vi "Get Interrupt Status.vi"(7 "I2C Channel":u8, 8 "error in (no error)":errorcluster, 11 "LINX Resource In":T1) -> (0 "error out":errorcluster, 1 "Raw Data Ready":bool, 2 "PLL Ready":bool, 3 "LINX Resource Out":T1)   [LabVIEW 2014, in "LMH-LINX.lvlib" / "ITG3200.lvlib"]
uses:
  <vilib>/MakerHub/LINX/Public/Sensors/Gyroscopes/ITG3200/ITG3200.lvlib
  <vilib>/MakerHub/LINX/Private/Type Defs/LINX Ref.ctl
  <vilib>/MakerHub/LINX/Private/Type Defs/Platform.ctl
  <vilib>/MakerHub/LINX/Private/Type Defs/Interface.ctl
  <vilib>/MakerHub/LINX/Private/Device/Type Defs/LINX Device Config.ctl
  <vilib>/MakerHub/LINX/Private/Device/Type Defs/TCP Config.ctl
  <vilib>/MakerHub/LINX/Private/Device/Type Defs/Channels.ctl
  <vilib>/MakerHub/LINX/Private/Local IO/LinxI2cWrite.vi
  <vilib>/MakerHub/LINX/Public/Utilities/Check Channel.vi
  <vilib>/MakerHub/LINX/Private/Utilties/Generate Error.vi
  <vilib>/MakerHub/LINX/LMH-LINX.lvlib
  <vilib>/MakerHub/LINX/Private/Device/Device.lvlib
panel:
  # "INPUTS"
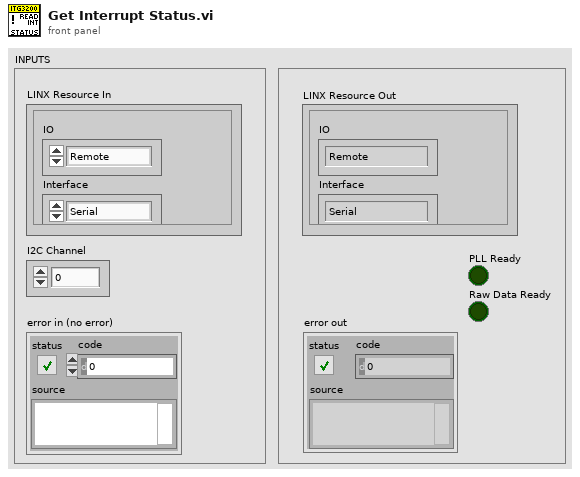
[diagram p1: front panel]
types:
  T1 = typedef "LMH-LINX.lvlib/LINX Ref.ctl" = cluster{"IO":T2, "Interface":T3, "LINX Device Config":T4}
  T2 = typedef "LMH-LINX.lvlib/Platform.ctl" = enum16{"Remote", "Local"}
  T3 = typedef "LMH-LINX.lvlib/Interface.ctl" = enum16{"Serial", "TCP"}
  T4 = typedef "LMH-LINX.lvlib/Device.lvlib/LINX Device Config.ctl" = cluster{"Interface":T3, "COM Port":refnum<visa-resource-name>, "TCP Configuration":T5, "Device Family":u8, "Device ID":u8, "Device Name":string, "TCP Ref":refnum<k5>, "Channels":T6}
  T5 = typedef "LMH-LINX.lvlib/Device.lvlib/TCP Config.ctl" = cluster{"IP Address":string, "Port":u16}
  T6 = typedef "LMH-LINX.lvlib/Channels.ctl" = cluster{"DI":u8[], "DO":u8[], "AI":u8[], "AO":u8[], "PWM":u8[], "QE":u8[], "UART":u8[], "I2C 2":u8[], "SPI":u8[], "CAN":u8[], "Servo":u8[], "AI Ref (V)":dbl, "AI Resolution (Bits)":u8, "AO Ref (V)":dbl, "AO Resolution (Bits)":u8}
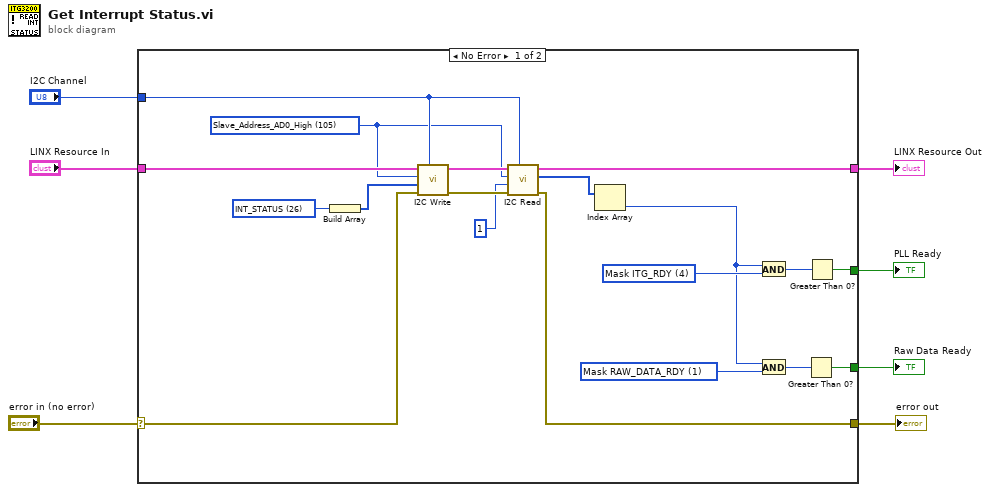
[diagram p0: block diagram]
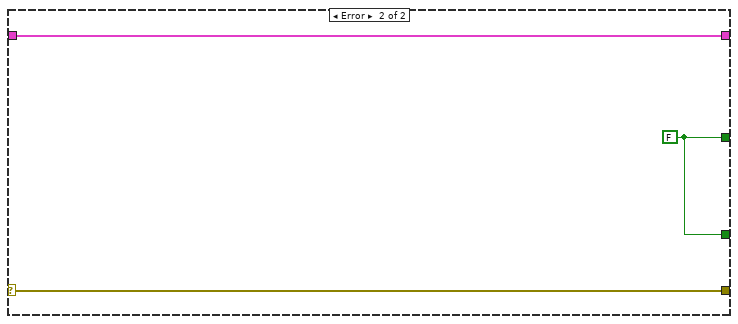
[diagram p2: hidden frame]
diagram:
  n1 = case shown="No Error" "error in (no error)" {
    selector: "error in (no error)" -> [w25 w29]
    tunnel: [w24 w29] -> w6
    tunnel: "LINX Resource In" -> [w26 w28]
    tunnel: "I2C Channel" -> [w22 _]
    tunnel: [w23 w28] -> w3
    tunnel: [w9 w27] -> w2
    tunnel: [w8 w27] -> w1
    frame No Error {
      w13 = u8 1 items=["Mask ITG_RDY"=4, "Mask RAW_DATA_RDY"=1] ("<INT STATUS> Register Masks")
      w14 = u8 4 items=["Mask ITG_RDY"=4, "Mask RAW_DATA_RDY"=1] ("<INT STATUS> Register Masks")
      w21 = u8 26 items=["WHO_AM_I"=0, "SMPLRT_DIV"=21, "DLPF_FS"=22, "INT_CFG"=23, "INT_STATUS"=26, "TEMP_OUT_H"=27, "TEMP_OUT_L"=28, "GYRO_XOUT_H"=29, "GYRO_XOUT_L"=30, "GYRO_YOUT_H"=31, "GYRO_YOUT_L"=32, "GYRO_ZOUT_H"=33, "GYRO_ZOUT_L"=34, "PWR_MGM"=62] ("Register Map")
      w17 = u8 105 items=["Slave_Address_AD0_Low"=104, "Slave_Address_AD0_High"=105] ("Slave Addresses")
      n2 = Build Array(w21) -> (w20:u8[])
      n3 = call <vilib>:"I2C Write.vi"("I2C Channel"=w22, "Error In"=w25, "Data"=w20, "I2C Slave Address (0)"=w17, "LINX Resource"=w26) -> ("Error Out"=w18:errorcluster, "LINX Resource"=w19:T1)  [unwired: 5 in]
      n4 = call <vilib>:"I2C Read.vi"("I2C Channel"=w22, "Error In"=w18, "Bytes To Read"=u8 1, "I2C Slave Address (0)"=w17, "LINX Resource"=w19) -> ("Error Out"=w24:errorcluster, "Data"=w15:u8[], "LINX Resource"=w23:T1)  [unwired: 4 in]
      n5 = Index Array(array=w15) -> (element=w12:u8)  [unwired: 1 in]
      n6 = And(x=w12, y=w14) -> (x .and. y?=w11:u8)
      n7 = And(x=w12, y=w13) -> (x .and. y?=w10:u8)
      n8 = Greater Than 0?(x=w10) -> (x > 0?=w8:bool)
      n9 = Greater Than 0?(x=w11) -> (x > 0?=w9:bool)
    }
    frame Error {
      w27 = FALSE
    }
  }
  "error out" <- w6
  "LINX Resource Out" <- w3
  "PLL Ready" <- w2
  "Raw Data Ready" <- w1
